vi "Channel Measurement Get S Parameter.vi"(8 "error in (no error)":errorcluster {"code" format="%.0x"}, 9 "RepCapIdentifier":string, 11 "instrument handle":refnum<k15>) -> (0 "error out":errorcluster {"code" format="%.0x"}, 1 "pSourcePortVal":i32, 2 "pReceiverPortVal":i32, 3 "instrument handle out":refnum<k15>)   [LabVIEW 2014, in "Agilent NA.lvlib"]
doc: "Returns the for Source port and Receiver port number specified in measurement"
uses:
  Agilent NA.lvlib
  AgNA.dll
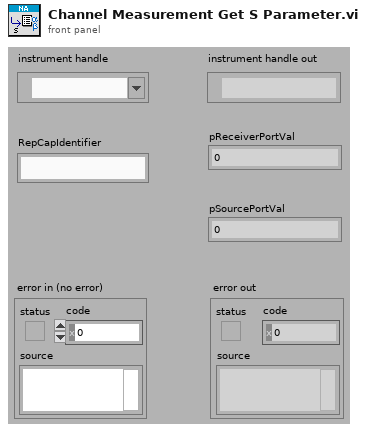
[diagram p1: front panel]
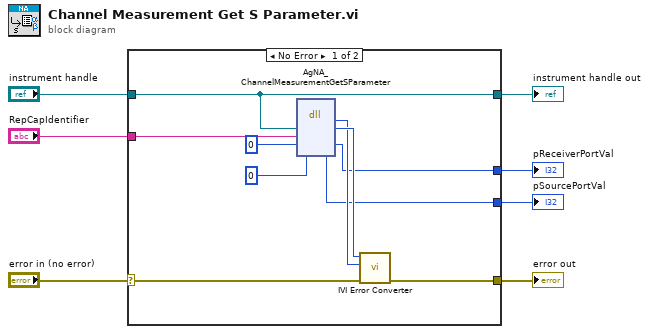
[diagram p0: block diagram]
diagram:
  n1 = case shown="No Error" "error in (no error)" {
    selector: "error in (no error)" -> [w15 w19]
    tunnel: [w14 w19] -> w7
    tunnel: "RepCapIdentifier" -> [w13 _]
    tunnel: [w11 _] -> w4
    tunnel: [w9 _] -> w3
    tunnel: [w8 w18] -> w2
    tunnel: "instrument handle" -> [w8 w18]
    frame No Error {
      n2 = dll-call lib="AgNA**.dll" fn="AgNA_ChannelMeasurementGetSParameter"("Vi"=w8, "RepCapIdentifier"=w13, "pReceiverPortVal"=0, "pSourcePortVal"=0) -> (w16:i32, "Vi"=w17:u32, "pReceiverPortVal"=w11:i32, "pSourcePortVal"=w9:i32)  [unwired: 4 in, 2 out]
      n3 = call "IVI Error Converter.vi"("error in (no error)"=w15, "IVI error code (0)"=w16, "instrument handle"=w17) -> ("error out"=w14:errorcluster)  [unwired: 7 in, 1 out]
    }
    frame Error {
    }
  }
  "error out" <- w7
  "instrument handle out" <- w2
  "pReceiverPortVal" <- w4
  "pSourcePortVal" <- w3
